vi "Modbus_Read_Sequential.vi"(5 "Number of Elements":i32, 7 "Start Address":u16, 8 "error in (no error)":errorcluster, 11 "TCP Network Connection in":refnum<k5>) -> (0 "error out":errorcluster, 2 "Array of Elements (RMS)":sgl[](array[numeric]), 3 "TCP Network Connection out":refnum<k5>)   [LabVIEW 2014]
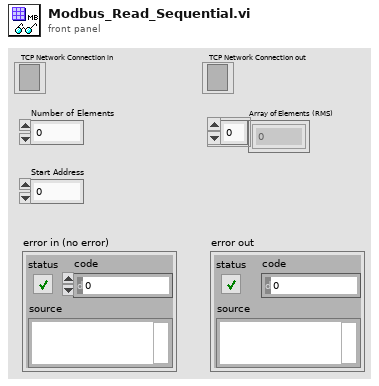
[diagram p1: front panel]
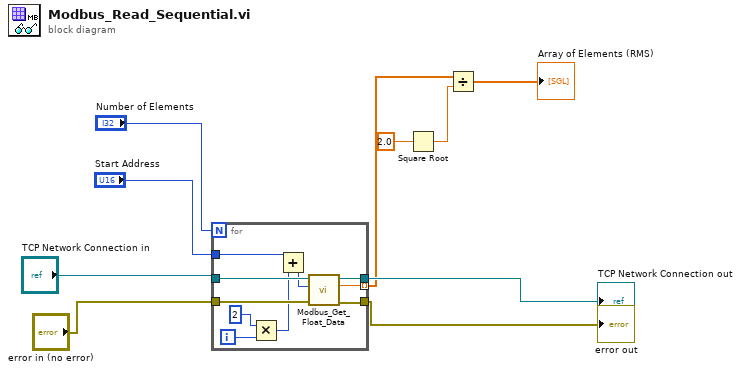
[diagram p0: block diagram]
diagram:
  n1 = for {
    N: "Number of Elements" -> [_]
    tunnel: "Start Address" -> [w13]
    tunnel: [w16] -> w7 mode=indexing
    tunnel: "TCP Network Connection in" -> [w20]
    tunnel: [w17] -> w9
    tunnel: "error in (no error)" -> [w19]
    tunnel: [w18] -> w10
    i -> [w15]
    n2 = Multiply(x=2, y=w15) -> (x*y=w12:i32)
    n3 = Add(x=w13, y=w12) -> (x+y=w11:i32)
    n4 = call "Modbus_Get_Float_Data.vi"("error in (no error)"=w19, "Starting Address (2 Bytes)"=w11, "TCP Network Connection in"=w20) -> ("error out"=w18:errorcluster, "Numeric"=w16:sgl, "TCP Network Connection out"=w17:refnum<k5>)  [unwired: 5 in, 1 out]
  }
  "error out" <- w10
  "TCP Network Connection out" <- w9
  n5 = Square Root(x=2.0) -> (sqrt(x)=w1:dbl)
  n6 = Divide(x=w7, y=w1) -> (x/y=→"Array of Elements (RMS)":dbl[])
